vi "Configure test.vi"(6 "Assert VI Path":path, 7 "Existing Queue Elements":string, 8 "error in (no error)":errorcluster, 11 "Basic Str Contains in":refnum<class "Str Contains.lvclass">) -> (0 "error out":errorcluster, 3 "Basic Str Contains out":refnum<class "Str Contains.lvclass">)   [LabVIEW 2018, in "Str Contains.lvclass"]
uses:
  Str Contains.lvclass
  3bf232ee-c641-4083-b1e2-b425091e7f4b.vi
  <vilib>/JDP Science/JSONtext/Find Item.vi
  3bf232ee-c641-4083-b1e2-b425091e7f4b.vi/036f7caf-fbb0-42e0-a909-729ac2b7bf84.vi
  3bf232ee-c641-4083-b1e2-b425091e7f4b.vi/a1bb99ef-928d-44c6-a614-62ba71bb245a.vi
  <vilib>/JDP Science/JSONtext/String Subset.vi
  Test Class String IDs.vi
  <vilib>/JDP Science/JSONtext/Parsing/Parse Full Path or Item Name.vi
  <vilib>/JDP Science/JSONtext/Offset/Find Item Locations by Path.vi
  <vilib>/JDP Science/JSONtext/JSON text to Variant.vi
  <vilib>/JDP Science/JSONtext/Variant to JSON Text.vi
  <vilib>/JDP Science/JSONtext/Set Item.vi
  String.lvclass
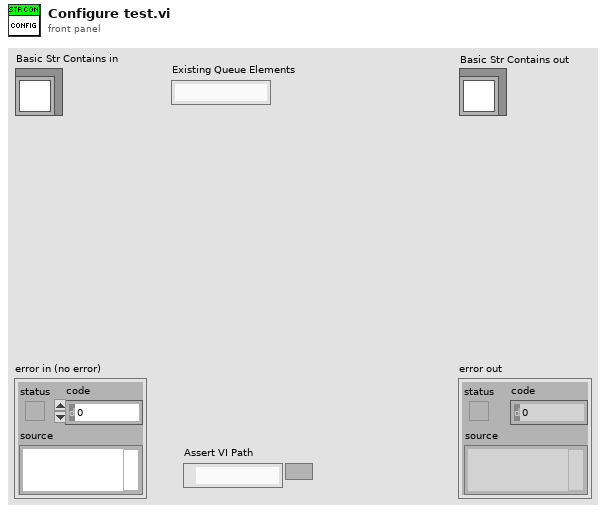
[diagram p1: front panel]
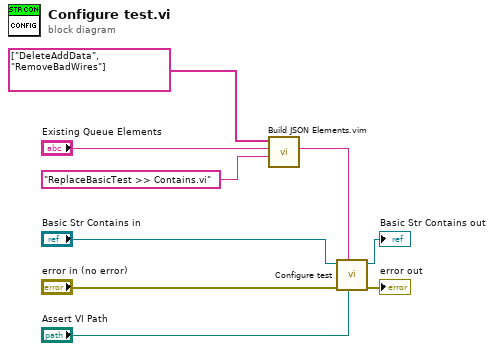
[diagram p0: block diagram]
diagram:
  n1 = call "Build JSON Elements.vim"("Append Element(s)"="ReplaceBasicTest >> Contains.vi", "JSON Elements in ({})"="Existing Queue Elements", "Prepend Element(s)"=string[] ["DeleteAddData", "RemoveBadWires"]) -> ("JSON Elements out"=w2:string)  [unwired: 8 in]
  n2 = call-parent "Configure test.vi"("Assert VI Path"="Assert VI Path", "Existing Queue Elements"=w2, "error in (no error)"="error in (no error)", "Basic String in"="Basic Str Contains in") -> ("error out"=→"error out":errorcluster, "Basic String out"=→"Basic Str Contains out":refnum<class "Str Contains.lvclass">)  [unwired: 6 in]
